vi "Connect to GoreAwsIotDev.vi"(8 "error in":errorcluster) -> (0 "error out":errorcluster, 2 "server certificate chain":cluster{"certificate":u8[]}[](array[cluster]), 3 "TCP Network Connection out":refnum<k5>)   [LabVIEW 2020]
uses:
  src/GoreAwsIot/AwsProvision.ctl
panel:
  out "error out 2":errorcluster
  out "TLS?":bool
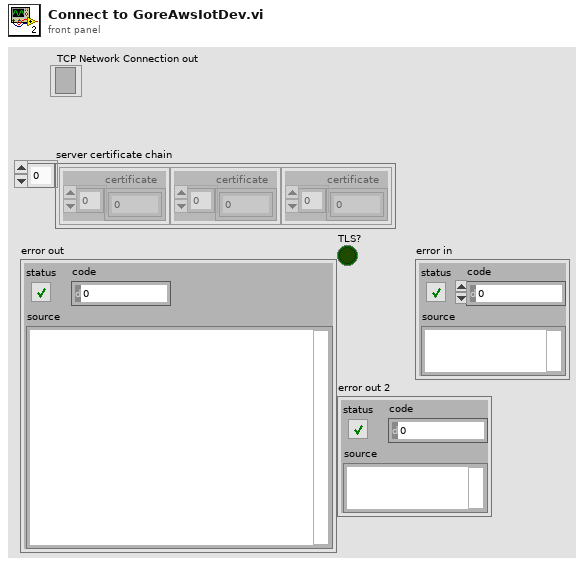
[diagram p1: front panel]
types:
  T1 = typedef "AwsProvision.ctl" = cluster{"device":cluster{"certificateArn":string, "certificateId":string, "certificatePem":string, "topic":string, "id":string, "keyPair":cluster{"PublicKey":string, "PrivateKey":string}}, "iotcore":cluster{"ca":string, "connectivity":cluster{"HostAddress":string}[]}}
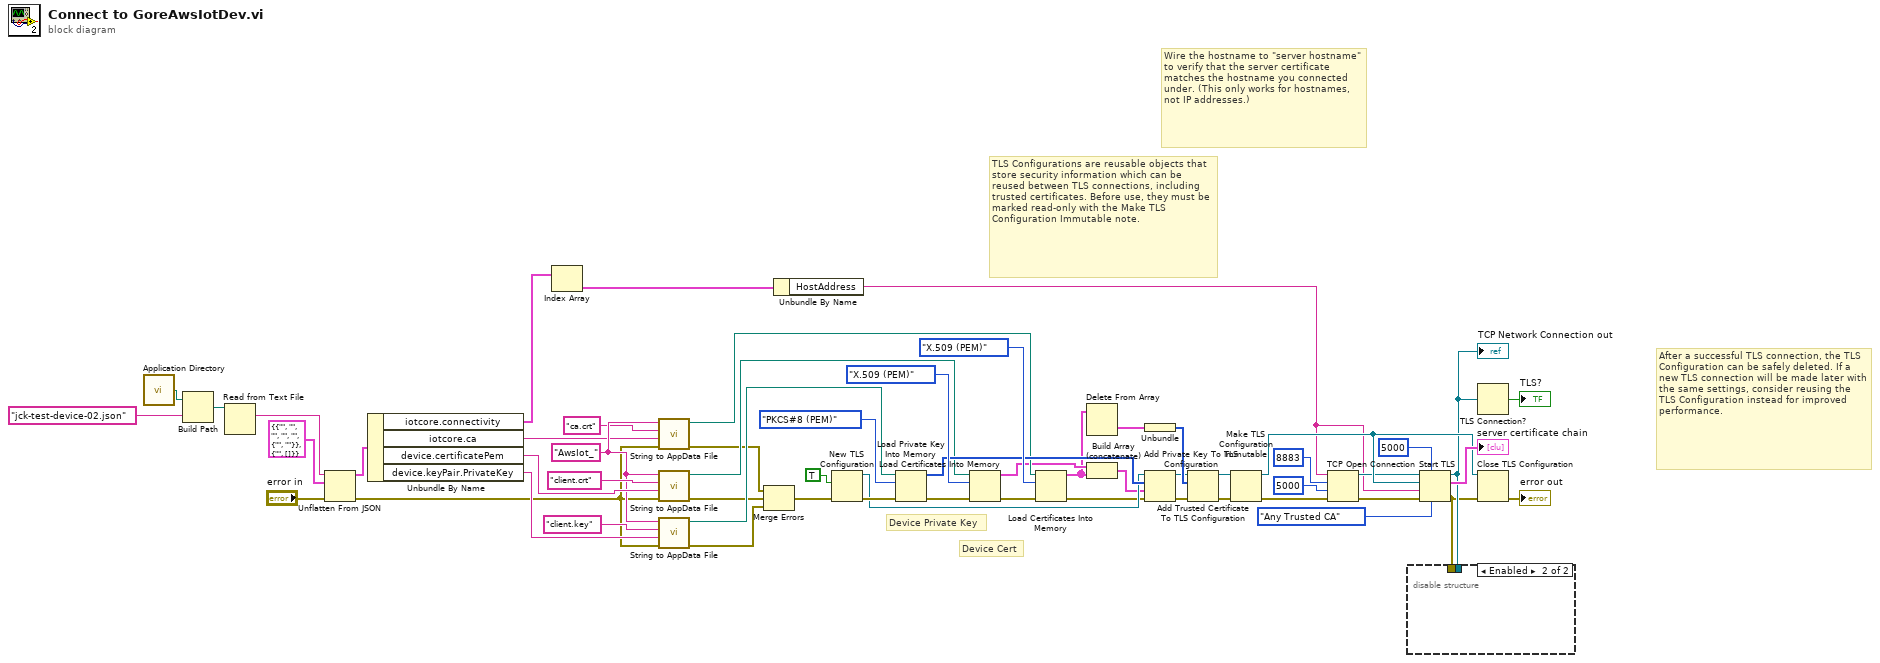
[diagram p0: block diagram]
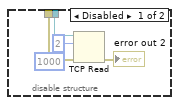
[diagram p2: hidden frame]
diagram:
  w19 = "AwsIot_" ("Hostname")
  # "Device Cert"
  # "Device Private Key"
  # "Wire the hostname to \"server hostname\" to verify that the server certificate matches the hostname you connected under. (This only works for hostnames, not IP addresses.)"
  # "TLS Configurations are reusable objects that store security information which can be reused between TLS connections, including trusted certificates. Before use, they must be marked read-only with the Make TLS Configuration Immutable note."
  # "After a successful TLS connection, the TLS Configuration can be safely deleted. If a new TLS connection will be made later with the same settings, consider reusing the TLS Configuration instead for improved performance."
  n1 = call <vilib>:"Application Directory.vi"() -> ("Application Directory"=w35:path)
  n2 = Build Path(base path=w35, name or relative path="jck-test-device-02.json") -> (appended path=w33:path)
  n3 = Read from Text File(file (use dialog)=w33) -> (text=w32:string)  [unwired: 3 in, 3 out]
  n4 = Unflatten From JSON(JSON string=w32, type and defaults=T1 {"device"={"certificateArn"="", "certificateId"="", "certificatePem"="", "topic"="", "id"="", "keyPair"={"PublicKey"="", "PrivateKey"=""}}, "iotcore"={"ca"="", "connectivity"=[]}} ("AwsProvision"), error in (no error)="error in") -> (value=w30:T1, error out=w13:errorcluster)  [unwired: 4 in]
  n5 = Unbundle By Name(w30) -> ("iotcore.connectivity"=w22:cluster{"HostAddress":string}[], "iotcore.ca"=w17:string, "device.certificatePem"=w26:string, "device.keyPair.PrivateKey"=w25:string)
  n6 = Index Array(array=w22) -> (element=w21:cluster{"HostAddress":string})  [unwired: 1 in]
  n7 = call "String to AppData File.vi"("error in"=w13, "Contents"=w17, "Filename"="ca.crt" ("Hostname"), "Prefix"=w19) -> ("error out"=w16:errorcluster, "path"=w29:path)  [unwired: 6 in]
  n8 = call "String to AppData File.vi"("error in"=w13, "Contents"=w26, "Filename"="client.crt" ("Hostname"), "Prefix"=w19) -> ("error out"=w15:errorcluster, "path"=w23:path)  [unwired: 6 in]
  n9 = call "String to AppData File.vi"("error in"=w13, "Contents"=w25, "Filename"="client.key" ("Hostname"), "Prefix"=w19) -> ("error out"=w14:errorcluster, "path"=w24:path)  [unwired: 6 in]
  n10 = Merge Errors(w16, w15, w14) -> (w12:errorcluster)
  n11 = Unbundle By Name(w21) -> ("HostAddress"=w1:string)
  n12 = New TLS Configuration(8:w12, 10:TRUE ("load OS trusted CAs?")) -> (0:w45:errorcluster, 3:w44:refnum<k36>)
  n13 = Load Private Key Into Memory(8:w45, 10:enum32{"PKCS#8 (PEM)", "PKCS#8 (DER)"}."PKCS#8 (PEM)" ("format"), 11:w24) -> (0:w10:errorcluster, 3:w46:u8[])  [unwired: 1 in]
  n14 = Load Certificates Into Memory(8:w10, 10:enum32{"X.509 (PEM)"}."X.509 (PEM)" ("format"), 11:w23) -> (0:w9:errorcluster, 3:w6:cluster{"certificate":u8[]}[])
  n15 = Load Certificates Into Memory(8:w9, 10:enum32{"X.509 (PEM)"}."X.509 (PEM)" ("format"), 11:w29) -> (0:w8:errorcluster, 3:w5:cluster{"certificate":u8[]}[])
  n16 = Delete From Array(array=w5) -> (deleted portion=w51:cluster{"certificate":u8[]})  [unwired: 2 in, 1 out]
  n17 = Build Array (concatenate)(w6, w5) -> (w4:cluster{"certificate":u8[]}[])
  n18 = Unbundle(w51) -> ("certificate"=w52:u8[])
  n19 = Add Private Key To TLS Configuration(8:w8, 9:w4, 10:w46, 11:w44) -> (0:w7:errorcluster, 3:w47:refnum<k36>)
  n20 = Add Trusted Certificate To TLS Configuration(8:w7, 10:w52, 11:w47) -> (0:w49:errorcluster, 3:w48:refnum<k36>)
  n21 = Make TLS Configuration Immutable(8:w49, 11:w48) -> (0:w36:errorcluster, 3:w40:refnum<k36>)
  n22 = TCP Open Connection(address=w1, remote port or service name=u16 8883 ("Port"), timeout ms (60000)=5000, error in (no error)=w36) -> (connection ID=w38:refnum<k5>, error out=w39:errorcluster)  [unwired: 1 in]
  n23 = Start TLS(6:enum32{"Any Trusted CA", "None"}."Any Trusted CA" ("server certificate validation"), 7:5000 ("timeout ms"), 8:w39, 9:w1, 10:w40, 11:w38) -> (0:w2:errorcluster, 2:→"server certificate chain":cluster{"certificate":u8[]}[], 3:w3:refnum<k5>)
  "TCP Network Connection out" <- w3
  n24 = disable-structure shown="Enabled" {
    disable-tunnel: w3 -> [w62 _]
    disable-tunnel: w2 -> [w61 _]
    frame Disabled {
      n25 = TCP Read(connection ID=w62, bytes to read=2, error in (no error)=w61, 9:1000 ("timeout ms (25000)")) -> (error out=→"error out 2":errorcluster)  [unwired: 1 in, 2 out]
    }
    frame Enabled {
    }
  }
  n26 = TLS Connection?(1:w3) -> (0:→"TLS?":bool)
  n27 = Close TLS Configuration(8:w2, 11:w40) -> (0:→"error out":errorcluster)
